vi "close.vi"(8 "error in":errorcluster, 11 "asynchronous execution module runtime In":refnum<class "asynchronous execution module runtime.lvclass">) -> (0 "error out":errorcluster)   [LabVIEW 2013, in "asynchronous execution module runtime.lvclass"]
doc: "Provides an interface for terminating a component instance. While this interface performs no operations, a child should close and deallocate any open references or memory."
uses:
  asynchronous execution module runtime.lvclass
  asynchronous execution module runtime.lvclass/asynchronous execution module runtime.ctl
  <vilib>/NI/Tag Bus Module Framework/runtime/TBM module execution interface.lvclass
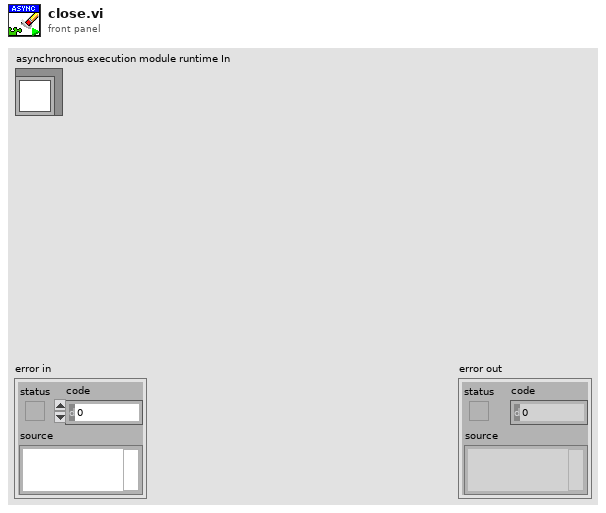
[diagram p1: front panel]
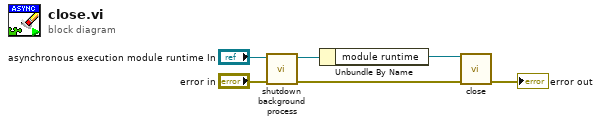
[diagram p0: block diagram]
diagram:
  n1 = call "shutdown background process.vi"("error in"="error in", "asynchronous execution module runtime In"="asynchronous execution module runtime In") -> ("error out"=w3:errorcluster, "asynchronous execution module runtime Out"=w4:refnum<class "asynchronous execution module runtime.lvclass">)  [unwired: 8 in]
  n2 = Unbundle By Name(w4) -> ("module runtime"=w1:refnum<class "TBM module execution interface.lvclass">)
  n3 = call-dynamic "close.vi"("error in"=w3, "module in"=w1) -> ("error out"=→"error out":errorcluster)  [unwired: 9 in]
